vi "exnFormulaBlock Ex_Inst_Formula.vi"(0 "X4":dynamicdata(graph), 1 "X3":dynamicdata(graph), 2 "X2":dynamicdata(graph), 3 "X1":dynamicdata(graph), 5 "X5":dynamicdata(graph), 7 "X6":dynamicdata(graph), 9 "X7":dynamicdata(graph), 11 "error in (no error)":errorcluster, 12 "X8":dynamicdata(graph)) -> (4 "Result":dynamicdata(graph), 15 "error out":errorcluster)   [LabVIEW 2020]
doc: "Uses a calculator interface to create mathematical formulas. You can use this Express VI to perform most math functions that a basic scientific calculator can compute."
panel:
  in  "Tab Control":T1(tab)
  in  "Name Modifier":string="Formula Result"
  in  "numinputs":dbl
  in  "Formula Output":string="X1"
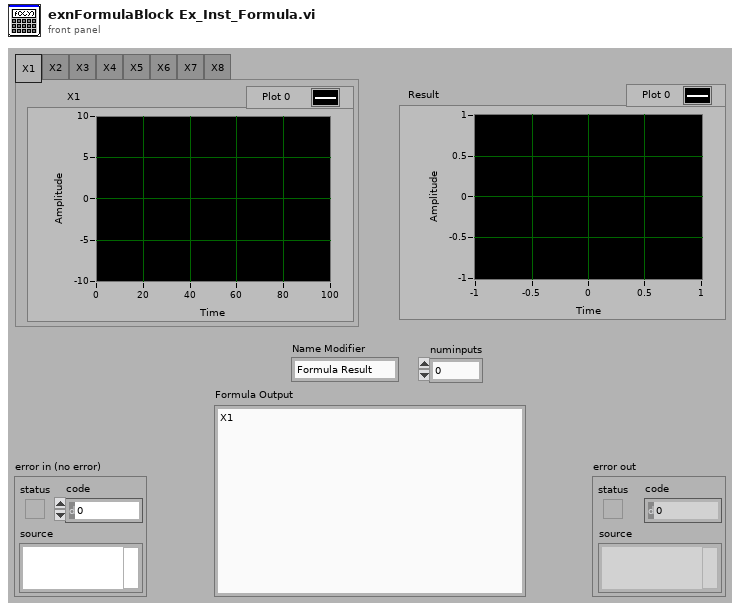
[diagram p1: front panel]
types:
  T1 = enum32{"X1", "X2", "X3", "X4", "X5", "X6", "X7", "X8"}
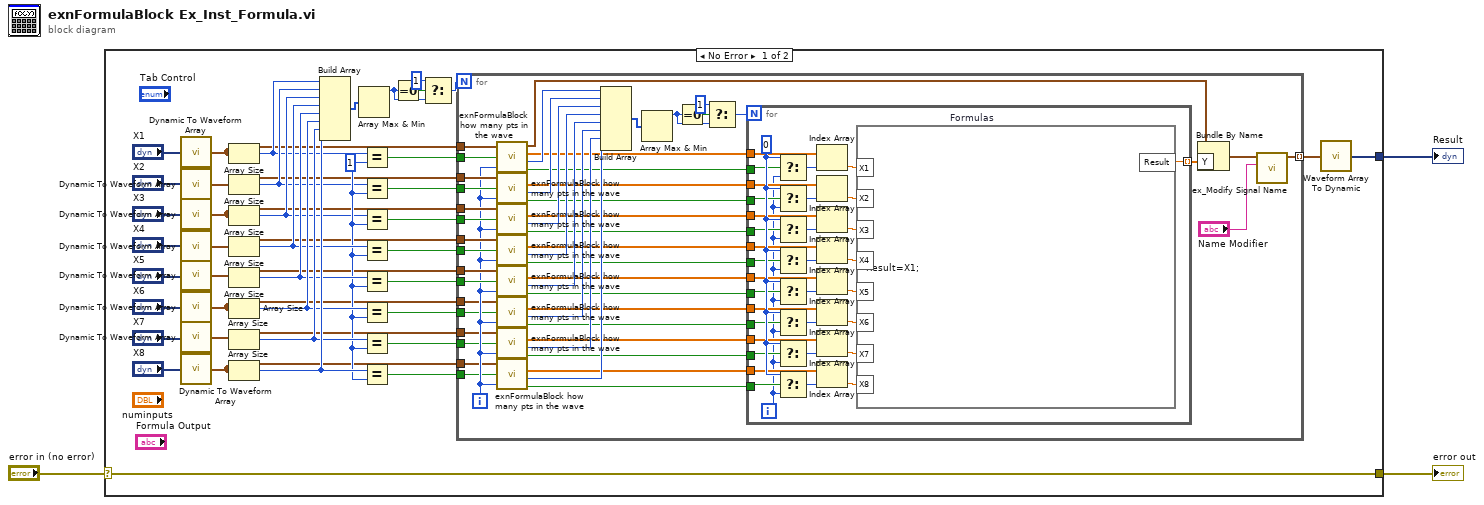
[diagram p0: block diagram]
diagram:
  n1 = case shown="No Error" "error in (no error)" {
    selector: "error in (no error)" -> [w4 w131]
    tunnel: [w12 _] -> w3
    tunnel: [w4 w131] -> w1
    frame No Error {
      w38 = u8 1 ("y")
      n2 = call <vilib>:"Dynamic To Waveform Array.vi"("Input"="X1") -> ("Output"=w20:waveform(dbl)[])  [unwired: 4 in]
      n3 = call <vilib>:"Dynamic To Waveform Array.vi"("Input"="X2") -> ("Output"=w11:waveform(dbl)[])  [unwired: 4 in]
      n4 = call <vilib>:"Dynamic To Waveform Array.vi"("Input"="X3") -> ("Output"=w10:waveform(dbl)[])  [unwired: 4 in]
      n5 = call <vilib>:"Dynamic To Waveform Array.vi"("Input"="X4") -> ("Output"=w9:waveform(dbl)[])  [unwired: 4 in]
      n6 = call <vilib>:"Dynamic To Waveform Array.vi"("Input"="X5") -> ("Output"=w8:waveform(dbl)[])  [unwired: 4 in]
      n7 = call <vilib>:"Dynamic To Waveform Array.vi"("Input"="X6") -> ("Output"=w7:waveform(dbl)[])  [unwired: 4 in]
      n8 = call <vilib>:"Dynamic To Waveform Array.vi"("Input"="X7") -> ("Output"=w6:waveform(dbl)[])  [unwired: 4 in]
      n9 = call <vilib>:"Dynamic To Waveform Array.vi"("Input"="X8") -> ("Output"=w5:waveform(dbl)[])  [unwired: 4 in]
      n10 = Array Size(array=w20) -> (size(s)=w35:i32)
      n11 = Array Size(array=w11) -> (size(s)=w36:i32)
      n12 = Array Size(array=w10) -> (size(s)=w37:i32)
      n13 = Array Size(array=w9) -> (size(s)=w39:i32)
      n14 = Array Size(array=w8) -> (size(s)=w40:i32)
      n15 = Array Size(array=w7) -> (size(s)=w41:i32)
      n16 = Array Size(array=w6) -> (size(s)=w42:i32)
      n17 = Array Size(array=w5) -> (size(s)=w43:i32)
      n18 = Build Array(w35, w36, w37, w39, w40, w41, w42, w43) -> (w34:i32[])
      n19 = Array Max & Min(array=w34) -> (max value=w24:i32)  [unwired: 3 out]
      n20 = Equal?(x=w35, y=w38) -> (x = y?=w33:bool)
      n21 = Equal?(x=w36, y=w38) -> (x = y?=w32:bool)
      n22 = Equal?(x=w37, y=w38) -> (x = y?=w31:bool)
      n23 = Equal?(x=w39, y=w38) -> (x = y?=w30:bool)
      n24 = Equal?(x=w40, y=w38) -> (x = y?=w29:bool)
      n25 = Equal?(x=w41, y=w38) -> (x = y?=w28:bool)
      n26 = Equal?(x=w42, y=w38) -> (x = y?=w27:bool)
      n27 = Equal?(x=w43, y=w38) -> (x = y?=w26:bool)
      n28 = Equal To 0?(x=w24) -> (x = 0?=w25:bool)
      n29 = Select(t=1, s=w25, f=w24) -> (s? t:f=w22:i32)
      n30 = for {
        N: w22 -> [_]
        tunnel: [w46] -> w44 mode=indexing
        tunnel: w33 -> [w92]
        tunnel: w32 -> [w89]
        tunnel: w31 -> [w86]
        tunnel: w30 -> [w83]
        tunnel: w29 -> [w79]
        tunnel: w28 -> [w74]
        tunnel: w27 -> [w73]
        tunnel: w26 -> [w72]
        tunnel: w20 -> [w90]
        tunnel: w11 -> [w87]
        tunnel: w10 -> [w84]
        tunnel: w9 -> [w81]
        tunnel: w8 -> [w80]
        tunnel: w7 -> [w75]
        tunnel: w6 -> [w76]
        tunnel: w5 -> [w77]
        i -> [w78]
        n31 = call <vilib>:"exnFormulaBlock how many pts in the wave.vi"("Array"=w90, "Boolean"=w92, "Iteration"=w78) -> ("Waveform"=w93:waveform(dbl), "Y"=w67:dbl[], "size(s)"=w91:i32, "x = y?"=w66:bool)
        n32 = call <vilib>:"exnFormulaBlock how many pts in the wave.vi"("Array"=w87, "Boolean"=w89, "Iteration"=w78) -> ("Y"=w65:dbl[], "size(s)"=w88:i32, "x = y?"=w64:bool)  [unwired: 1 out]
        n33 = call <vilib>:"exnFormulaBlock how many pts in the wave.vi"("Array"=w84, "Boolean"=w86, "Iteration"=w78) -> ("Y"=w63:dbl[], "size(s)"=w85:i32, "x = y?"=w62:bool)  [unwired: 1 out]
        n34 = call <vilib>:"exnFormulaBlock how many pts in the wave.vi"("Array"=w81, "Boolean"=w83, "Iteration"=w78) -> ("Y"=w61:dbl[], "size(s)"=w82:i32, "x = y?"=w55:bool)  [unwired: 1 out]
        n35 = call <vilib>:"exnFormulaBlock how many pts in the wave.vi"("Array"=w80, "Boolean"=w79, "Iteration"=w78) -> ("Y"=w60:dbl[], "size(s)"=w71:i32, "x = y?"=w59:bool)  [unwired: 1 out]
        n36 = call <vilib>:"exnFormulaBlock how many pts in the wave.vi"("Array"=w75, "Boolean"=w74, "Iteration"=w78) -> ("Y"=w58:dbl[], "size(s)"=w70:i32, "x = y?"=w54:bool)  [unwired: 1 out]
        n37 = call <vilib>:"exnFormulaBlock how many pts in the wave.vi"("Array"=w76, "Boolean"=w73, "Iteration"=w78) -> ("Y"=w57:dbl[], "size(s)"=w69:i32, "x = y?"=w53:bool)  [unwired: 1 out]
        n38 = call <vilib>:"exnFormulaBlock how many pts in the wave.vi"("Array"=w77, "Boolean"=w72, "Iteration"=w78) -> ("Y"=w56:dbl[], "size(s)"=w68:i32, "x = y?"=w52:bool)  [unwired: 1 out]
        n39 = Build Array(w91, w88, w85, w82, w71, w70, w69, w68) -> (w94:i32[])
        n40 = Array Max & Min(array=w94) -> (max value=w49:i32)  [unwired: 3 out]
        n41 = Equal To 0?(x=w49) -> (x = 0?=w51:bool)
        n42 = Select(t=u8 1, s=w51, f=w49) -> (s? t:f=w48:i32)
        n43 = for {
          N: w48 -> [_]
          tunnel: [w130] -> w95 mode=indexing
          tunnel: w67 -> [w119]
          tunnel: w66 -> [w118]
          tunnel: w65 -> [w117]
          tunnel: w64 -> [w116]
          tunnel: w63 -> [w115]
          tunnel: w62 -> [w114]
          tunnel: w61 -> [w113]
          tunnel: w60 -> [w112]
          tunnel: w59 -> [w111]
          tunnel: w58 -> [w110]
          tunnel: w57 -> [w109]
          tunnel: w56 -> [w108]
          tunnel: w55 -> [w107]
          tunnel: w54 -> [w106]
          tunnel: w53 -> [w105]
          tunnel: w52 -> [w97]
          i -> [w96]
          w129 = 0 ("t")
          n44 = Select(t=w129, s=w118, f=w96) -> (s? t:f=w125:i32)
          n45 = Select(t=w129, s=w116, f=w96) -> (s? t:f=w124:i32)
          n46 = Select(t=w129, s=w114, f=w96) -> (s? t:f=w123:i32)
          n47 = Select(t=w129, s=w107, f=w96) -> (s? t:f=w122:i32)
          n48 = Select(t=w129, s=w111, f=w96) -> (s? t:f=w121:i32)
          n49 = Select(t=w129, s=w106, f=w96) -> (s? t:f=w126:i32)
          n50 = Select(t=w129, s=w105, f=w96) -> (s? t:f=w127:i32)
          n51 = Select(t=w129, s=w97, f=w96) -> (s? t:f=w128:i32)
          n52 = Index Array(array=w119, index=w125) -> (element=w120:dbl)
          n53 = Index Array(array=w117, index=w124) -> (element=w104:dbl)
          n54 = Index Array(array=w115, index=w123) -> (element=w103:dbl)
          n55 = Index Array(array=w113, index=w122) -> (element=w102:dbl)
          n56 = Index Array(array=w112, index=w121) -> (element=w101:dbl)
          n57 = Index Array(array=w110, index=w126) -> (element=w100:dbl)
          n58 = Index Array(array=w109, index=w127) -> (element=w99:dbl)
          n59 = Index Array(array=w108, index=w128) -> (element=w98:dbl)
          n60 = formula code="Result=X1;" "Formulas"("X1"=w120, "X2"=w104, "X3"=w103, "X4"=w102, "X5"=w101, "X6"=w100, "X7"=w99, "X8"=w98) -> ("Result"=w130:dbl)
        }
        n61 = Bundle By Name(cluster=w93, "Y"=w95) -> (w47:waveform(dbl))
        n62 = call <vilib>:"ex_Modify Signal Name.vi"("Name Modifier"="Name Modifier", "waveform in"=w47) -> ("waveform out"=w46:waveform(dbl))  [unwired: 8 in, 1 out]
      }
      n63 = call <vilib>:"Waveform Array To Dynamic.vi"("Input"=w44) -> ("Output"=w12:dynamicdata)  [unwired: 4 in]
    }
    frame Error {
    }
  }
  "Result" <- w3
  "error out" <- w1
